vi "SG Filter (DVR).vi"(8 "error in":errorcluster, 10 "side points":i32, 11 "Data Value Reference in":refnum<data-value>) -> (0 "error out":errorcluster, 3 "Data Value Reference out":refnum<data-value>)   [LabVIEW 2016, in "Retrieve and Visualize.lvclass"]
uses:
  Retrieve and Visualize.lvclass
  <userlib>/LevyLab/XY Utilities/subVIs/Savitsky Golay Filter (multiple).vi
  <userlib>/LevyLab/XY Utilities/xy_utilities.lvlib
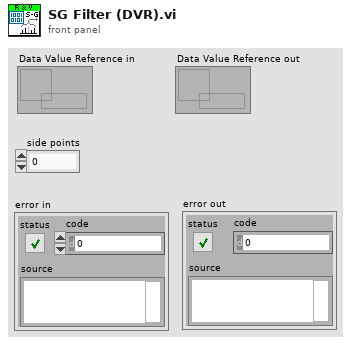
[diagram p1: front panel]
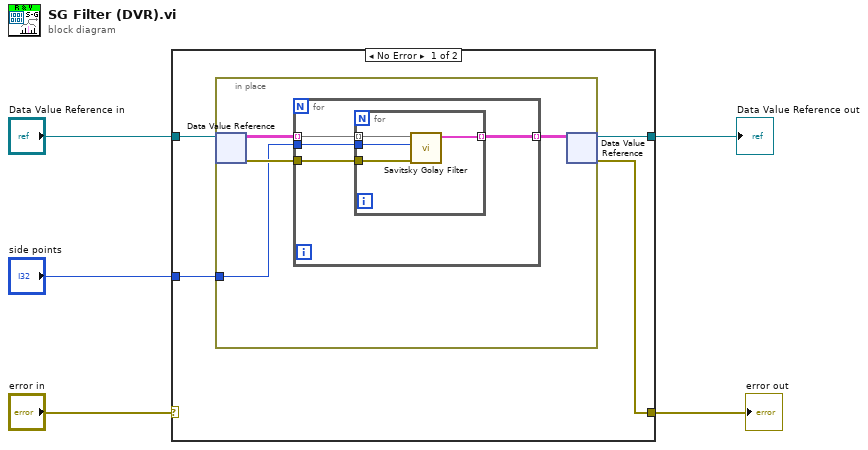
[diagram p0: block diagram]
diagram:
  n1 = case shown="No Error" "error in" {
    selector: "error in" -> [_ w23]
    tunnel: "side points" -> [w9 _]
    tunnel: [w8 w22] -> w4
    tunnel: "Data Value Reference in" -> [w7 w22]
    tunnel: [w6 w23] -> w2
    frame No Error {
      n2 = in-place {
        in-place-border: w9 -> [w10]
        n3 = in-place-dvr #1(w7) -> (w13:cluster{dbl[], dbl[]}[][][], w11:errorcluster)
        n4 = for {
          tunnel: [w17] -> w12 mode=indexing
          tunnel: w10 -> [w16]
          tunnel: w13 -> [w15] mode=indexing
          tunnel: w11 -> [w14]
          n5 = for {
            tunnel: [w20] -> w17 mode=indexing
            tunnel: w16 -> [w21]
            tunnel: w15 -> [w19] mode=indexing
            tunnel: w14 -> [w18]
            n6 = call-poly <userlib>:"Savitsky Golay Filter.vi"("error in (no error)"=w18, "side points"=w21, "XY-data"=w19) -> ("XY-data out"=w20:cluster{"X-array":dbl[], "Y-array":dbl[]}[])  [unwired: 7 in, 1 out]
          }
        }
        n7 = in-place-dvr #1(w12) -> (w8:refnum<data-value>, w6:errorcluster)
      }
    }
    frame Error {
    }
  }
  "Data Value Reference out" <- w4
  "error out" <- w2
